vi "Finish.vi"(8 "error in (no error)":errorcluster, 11 "Trace Controller in":refnum<class "Trace Controller.lvclass">) -> (0 "error out":errorcluster, 3 "Trace Controller out":refnum<class "Trace Controller.lvclass">)   [LabVIEW 2014, in "Robot Actor Framework.lvlib" / "Trace.lvlib" / "Trace Controller.lvclass"]
uses:
  Trace Controller.lvclass
  Trace Controller.lvclass/Trace Controller.ctl
  System Actor/System Actor Class/System Actor.lvclass
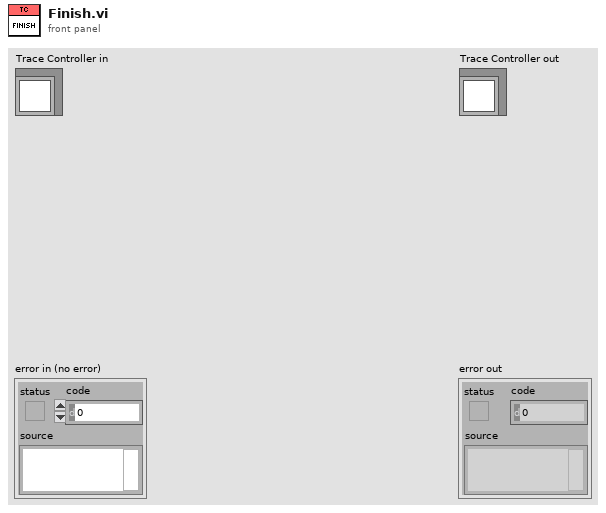
[diagram p1: front panel]
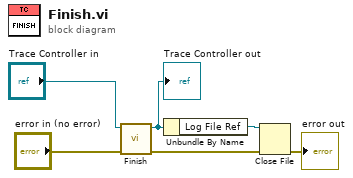
[diagram p0: block diagram]
diagram:
  n1 = call-parent "Finish.vi"("error in (no error)"="error in (no error)", "System Actor in"="Trace Controller in") -> ("error out"=w3:errorcluster, "System Actor out"=w5:refnum<class "Trace Controller.lvclass">)  [unwired: 8 in]
  "Trace Controller out" <- w5
  n2 = Unbundle By Name(w5) -> ("Log File Ref"=w1:refnum<file>)
  n3 = Close File(refnum=w1, error in=w3) -> (error out=→"error out":errorcluster)  [unwired: 1 out]
